vi "Is CSM Module - WhileLoop.vi"(8 "error in (no error)":errorcluster, 11 "WhileLoop in":refnum<vi>) -> (0 "error out":errorcluster, 1 "CSMType":T1, 2 "Is CSM Module?":bool, 3 "CSM Basic Refs":T2)   [LabVIEW 2017, in "CSM-Helper Utility.lvlib"]
doc: "#### Is CSM Module - WhileLoop.vi\n\nDetermine if it is a CSM module through While Loop reference\n\n-- <b>Controls</b> --\n- <b>WhileLoop</b>: While Loop reference\n\n-- <b>Indicators</b> --\n- <b>Is CSM Module?</b>: True If it is a CSM module\n- <b>CSM Basic Refs</b>: If This is a CSM module, It will return the basic references"
uses:
  CSM-Helper Utility.lvlib
  CSM Basic Refs.ctl
  CSM Module Type.ctl
  _Support/Relationship.llb/csmHelper-Relationship.lvlib
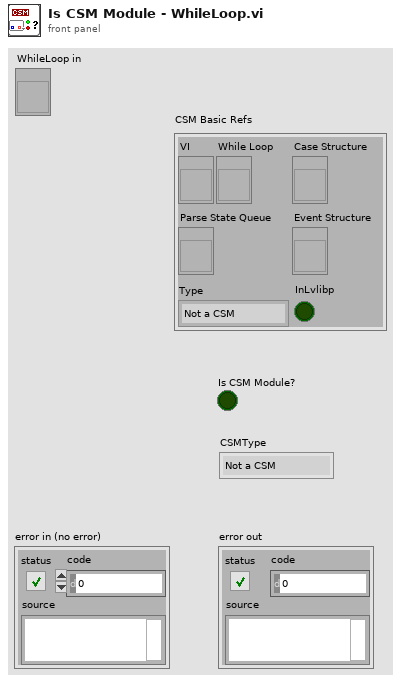
[diagram p1: front panel]
types:
  T1 = typedef "CSM-Helper Utility.lvlib/CSM Module Type.ctl" = enum16{"Not a CSM", "JKISM", "CSM"}
  T2 = typedef "CSM-Helper Utility.lvlib/CSM Basic Refs.ctl" = cluster{"VI":refnum<vi>, "While Loop":refnum<vi>, "Case Structure":refnum<vi>, "Parse State Queue":refnum<vi>, "Event Structure":refnum<vi>, "Type":T1, "InLvlibp":bool}
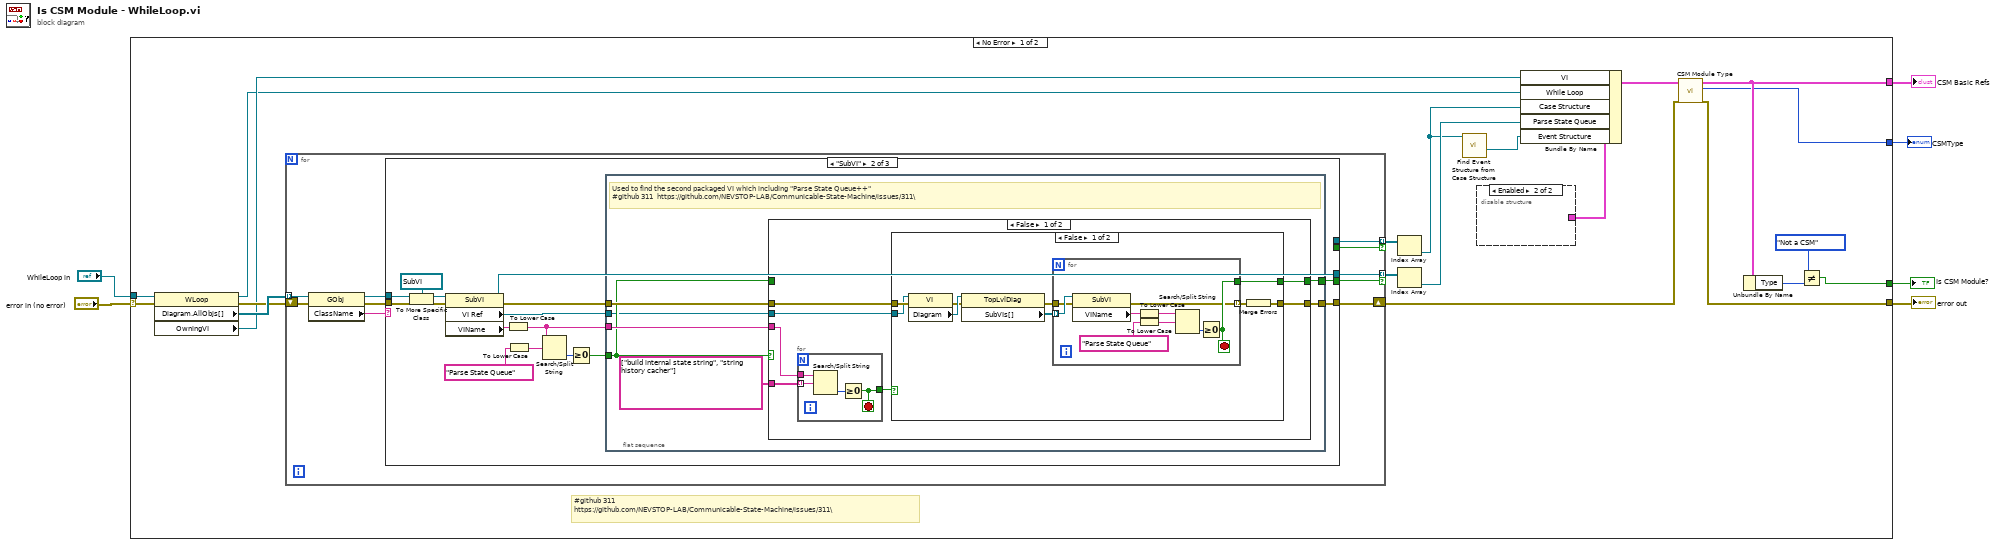
[diagram p0: block diagram]
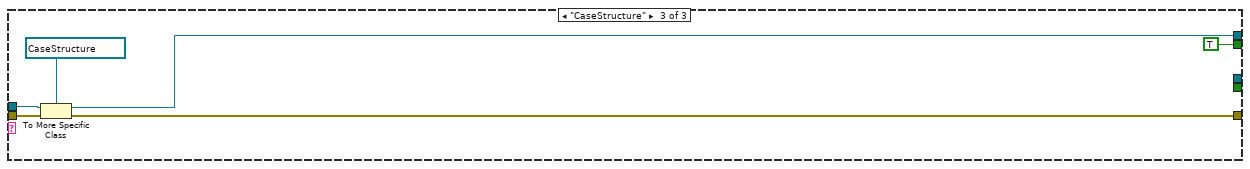
[diagram p5: hidden frame]
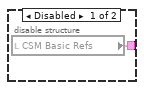
[diagram p6: hidden frame]
diagram:
  n1 = case shown="No Error" "error in (no error)" {
    selector: "error in (no error)" -> [w26 w100]
    tunnel: "WhileLoop in" -> [w22 _]
    tunnel: [w12 w100] -> w4
    tunnel: [w8 _] -> w3
    tunnel: [w11 _] -> w2
    tunnel: [w7 _] -> w1
    frame No Error {
      # "#github 311 \nhttps://github.com/NEVSTOP-LAB/Communicable-State-Machine/issues/311\\"
      n2 = property on="Property Node" class="WLoop"(reference=w22, error in=w26) -> (reference out=w18:refnum<vi>, error out=w24:errorcluster, "Diagram.AllObjs[]"=w25:refnum<vi>[], "OwningVI"=w19:refnum<vi>)
      n3 = for {
        tunnel: w25 -> [w36] mode=indexing
        shift-right: [w31] -> w13
        shift-left: w24 -> [w32]
        tunnel: [w30] -> w21 mode=indexing if=w27
        tunnel: [w29] -> w23 mode=indexing if=w28
        n4 = property class="GObj"(reference=w36, error in=w32) -> (reference out=w34:refnum<vi>, error out=w33:errorcluster, "ClassName"=w35:string)
        n5 = case shown="\"SubVI\"" w35 {
          tunnel: w34 -> [_ w52 w97]
          tunnel: w33 -> [w37 w51 w96]
          tunnel: [w37 w42 w95] -> w31
          tunnel: [_ w47 _] -> w30
          tunnel: [_ _ w94] -> w29
          tunnel: [_ _ TRUE] -> w28
          tunnel: [_ w40 _] -> w27
          frame Default {
          }
          frame "SubVI" {
            n6 = To More Specific Class(target class=refnum<vi> refnum ("SubVI Refnum"), reference=w52, error in=w51) -> (specific class reference=w50:refnum<vi>, error out=w49:errorcluster)
            n7 = property class="SubVI"(reference=w50, error in=w49) -> (reference out=w47:refnum<vi>, error out=w43:errorcluster, "VI Ref"=w38:refnum<vi>, "VIName"=w44:string)
            n8 = To Lower Case(string=w44) -> (all lower case string=w41:string)
            n9 = To Lower Case(string="Parse State Queue" ("VI Name")) -> (all lower case string=w46:string)
            n10 = Search/Split String(string=w41, search string/char (-)=w46) -> (offset of match=w45:i32)  [unwired: 1 in, 2 out]
            n11 = Greater Or Equal To 0?(x=w45) -> (x >= 0?=w39:bool)
            n12 = flat-sequence {
              tunnel: w43 -> [w60]
              tunnel: [w59] -> w42
              tunnel: w41 -> [w58]
              tunnel: [w57] -> w40
              tunnel: w39 -> [w56]
              tunnel: w38 -> [w55]
              frame #0 {
                # "Used to find the second packaged VI which including \"Parse State Queue++\"\n#github 311  https://github.com/NEVSTOP-LAB/Communicable-State-Machine/issues/311\\"
                n13 = case shown="False" w56 {
                  tunnel: w60 -> [w65 w92]
                  tunnel: [w64 w92] -> w59
                  tunnel: w58 -> [w66 _]
                  tunnel: string[] ["build internal state string", "string history cacher"] ("all lower case string") -> [w67 _]
                  tunnel: [w62 w91] -> w57
                  tunnel: w56 -> [_ w91]
                  tunnel: w55 -> [w63 _]
                  frame False {
                    n14 = for {
                      tunnel: w67 -> [w70] mode=indexing
                      tunnel: w66 -> [w71]
                      tunnel: [w68] -> w61
                      stop <- w68 stop-if-true
                      n15 = Search/Split String(string=w71, search string/char (-)=w70) -> (offset of match=w69:i32)  [unwired: 1 in, 2 out]
                      n16 = Greater Or Equal To 0?(x=w69) -> (x >= 0?=w68:bool)
                    }
                    n17 = case shown="False" w61 {
                      tunnel: w65 -> [w75 w90]
                      tunnel: [w79 w90] -> w64
                      tunnel: w63 -> [w74 _]
                      tunnel: [w72 _] -> w62
                      frame False {
                        n18 = property class="VI"(reference=w74, error in=w75) -> (error out=w77:errorcluster, "Diagram"=w78:refnum<vi>)  [unwired: 1 out]
                        n19 = property class="TopLvlDiag"(reference=w78, error in=w77) -> (error out=w76:errorcluster, "SubVIs[]"=w73:refnum<vi>[])  [unwired: 1 out]
                        n20 = for {
                          tunnel: w73 -> [w89] mode=indexing
                          tunnel: w76 -> [w88]
                          tunnel: [w82] -> w72
                          tunnel: [w81] -> w80 mode=indexing
                          stop <- w82 stop-if-true
                          n21 = property class="SubVI"(reference=w89, error in=w88) -> (error out=w81:errorcluster, "VIName"=w87:string)  [unwired: 1 out]
                          n22 = To Lower Case(string=w87) -> (all lower case string=w85:string)
                          n23 = To Lower Case(string="Parse State Queue" ("VI Name")) -> (all lower case string=w83:string)
                          n24 = Search/Split String(string=w85, search string/char (-)=w83) -> (offset of match=w86:i32)  [unwired: 1 in, 2 out]
                          n25 = Greater Or Equal To 0?(x=w86) -> (x >= 0?=w82:bool)
                        }
                        n26 = Merge Errors(w80) -> (w79:errorcluster)
                      }
                      frame True {
                      }
                    }
                  }
                  frame True {
                  }
                }
              }
            }
          }
          frame "CaseStructure" {
            n27 = To More Specific Class(target class=refnum<vi> refnum ("CaseSel Refnum"), reference=w97, error in=w96) -> (specific class reference=w94:refnum<vi>, error out=w95:errorcluster)
          }
        }
      }
      n28 = Index Array(array=w23) -> (element=w16:refnum<vi>)  [unwired: 1 in]
      n29 = Index Array(array=w21) -> (element=w17:refnum<vi>)  [unwired: 1 in]
      n30 = call "Find Event Structure from Case Structure.vi"("CaseStructure"=w16) -> ("EvntStruct Refnum"=w15:refnum<vi>)  [unwired: 9 in, 1 out]
      n31 = disable-structure shown="Enabled" {
        disable-tunnel: [w99 _] -> w20
        frame Disabled {
          n32 = local read "CSM Basic Refs"() -> (w99:T2)
        }
        frame Enabled {
        }
      }
      n33 = Bundle By Name(cluster=w20, "VI"=w19, "While Loop"=w18, "Case Structure"=w16, "Parse State Queue"=w17, "Event Structure"=w15) -> (w14:T2)
      n34 = call "CSM Module Type.vi"("Error in"=w13, "CSM Basic Refs"=w14) -> ("error out"=w12:errorcluster, "CSMType"=w7:T1, "CSM Basic Refs (dup)"=w11:T2)  [unwired: 7 in]
      n35 = Unbundle By Name(w11) -> ("Type"=w10:T1)
      n36 = Not Equal?(x=CSM_Module_Type."Not a CSM", y=w10) -> (x != y?=w8:bool)
    }
    frame Error {
    }
  }
  "error out" <- w4
  "CSM Basic Refs" <- w2
  "Is CSM Module?" <- w3
  "CSMType" <- w1
